vi "FlattenToDisplayString.vi"(8 "error in (no error)":errorcluster, 11 "FTPConfig in":refnum<class "FTPConfig.lvclass">) -> (0 "error out":errorcluster, 2 "String":string, 3 "FTPConfig out":refnum<class "FTPConfig.lvclass">)   [LabVIEW 2017, in "FileSync -- FTP.lvlib" / "FTPConfig.lvclass"]
uses:
  FTPConfig.lvclass
  FTPConfig.lvclass/FTPConfig.ctl
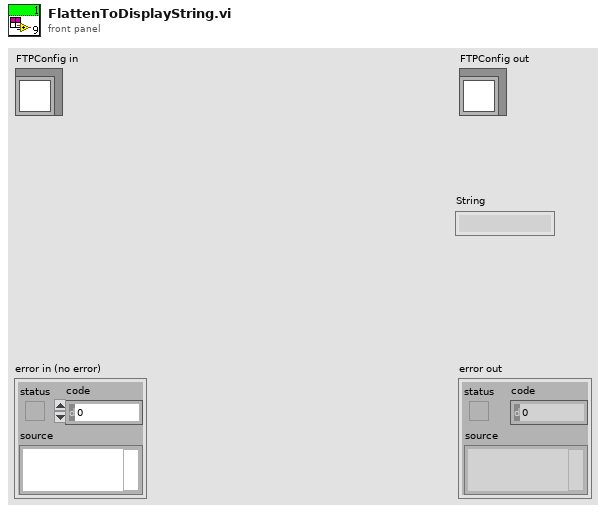
[diagram p1: front panel]
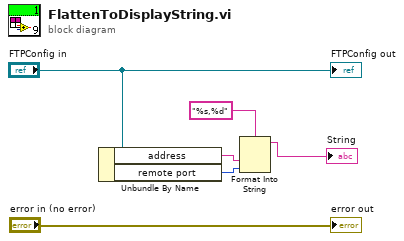
[diagram p0: block diagram]
diagram:
  n1 = Unbundle By Name("FTPConfig in") -> ("address"=w4:string, "remote port"=w3:u16)
  n2 = Format Into String(format string="%s,%d", w4, w3) -> (resulting string=→"String":string)  [unwired: 2 in, 1 out]
  "error out" <- "error in (no error)"
  "FTPConfig out" <- "FTPConfig in"
